vi "ROI_positions_UPDATE.vi"(1 "XY new position":dbl[](array[numeric]), 2 "XY positions IN":dbl[][](array[numeric])) -> (0 "XY positions OUT":dbl[][](array[numeric]))   [LabVIEW 2015]
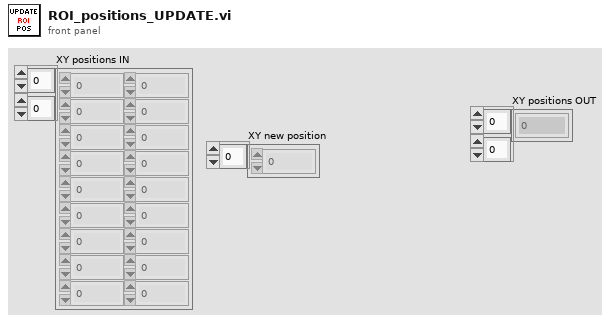
[diagram p1: front panel]
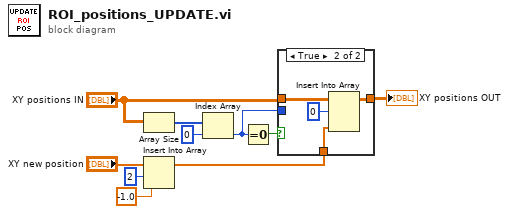
[diagram p0: block diagram]
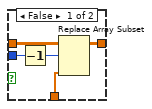
[diagram p2: hidden frame]
diagram:
  n1 = Array Size(array="XY positions IN") -> (size(s)=w7:i32[])
  n2 = Insert Into Array(array="XY new position", index=2, new element=-1.0 ("new element/subarray")) -> (w1:dbl[])
  n3 = Index Array(array=w7, index=0) -> (element=w10:i32)
  n4 = Equal To 0?(x=w10) -> (x = 0?=w9:bool)
  n5 = case shown="True" w9 {
    tunnel: "XY positions IN" -> [w15 w19]
    tunnel: w1 -> [w13 w17]
    tunnel: [w14 w16] -> w5
    tunnel: w10 -> [w12 _]
    frame False {
      n6 = Decrement(x=w12) -> (x-1=w11:i32)
      n7 = Replace Array Subset(array=w15, new element=w13, index (row)=w11) -> (w14:dbl[][])  [unwired: 1 in]
    }
    frame True {
      n8 = Insert Into Array(array=w19, index (row)=0, new element=w17) -> (w16:dbl[][])  [unwired: 1 in]
    }
  }
  "XY positions OUT" <- w5
